vi "PingPong.BRAMStorage.vi"(5 "Bank 1":refnum<k21>, 6 "Line Status In":T2, 7 "Bank 0":refnum<k21>, 8 "BRAM Bank0 Write?":bool, 9 "Read Info":cluster{"Read Address":u16, "Read Valid":bool}, 10 "Write Info":cluster{"Write Address":u16, "Write Valid":bool}, 11 "Frame Data In":T3={"Pixel Data"=[0, 0, 0, 0], "Timestamps"={"Frame Timestamp"=0, "Acq Trigger Timestamp"=0, "Next Trigger Timestamp"=0}}) -> (0 "Output Valid":bool, 1 "Line Status Out":T2, 3 "Data Out":i16[](array[numeric]))   [LabVIEW 2014]
uses:
  Acquisition Engine/Acquisition Status.ctl
  <vilib>/rvi/DataTransferAndStorage/Container/Common/niFpgaContainerExecOnDevCompGetState.vi
  <vilib>/rvi/Emulation/niFpgaEmulationIsFPGAContextNoSignature.vi
  <vilib>/rvi/DataTransferAndStorage/Container/Common/niFpgaContainerGetUniqueNameForEmu.vi
  <vilib>/rvi/Emulation/niFpgaProcessEmulError.vi
  <vilib>/rvi/Emulation/niFpgaSctlEmulationGetInTimedLoop.vi
  <vilib>/rvi/errors/nirviReportUnexpectedCaseInternalError (U32).vi
  <vilib>/rvi/Memory/Memory_Emulation/niFpgaMemoryEmulationCacheClearOnFirstRun.vi
  <vilib>/rvi/Memory/Memory_Emulation/nirvimemoryEmulationManagerCache_MakeExclusive.vi
  <vilib>/rvi/Memory/Memory_Emulation/niFpgaMemoryEmulationValidateCache.vi
  <vilib>/rvi/Memory/Memory_Emulation/nirvimemoryEmulationManagerCache_InsertValue.vi
  <vilib>/Utility/error.llb/Clear Errors.vi
  <vilib>/rvi/Memory/Memory_Emulation/nirvimemoryEmulationManagerCache_ReleaseExclusive.vi
  <vilib>/rvi/Memory/Memory_Emulation/nirvimemoryEmulationManagerCache_GetValue.vi
  <vilib>/rvi/Memory/Memory_Emulation/nirvimemoryEmulationManagerCache_SetValue.vi
  <vilib>/rvi/Emulation/niFpgaSctlEmulationResourceMgr.vi
  <vilib>/rvi/DataTransferAndStorage/Container/XNode/niFpgaContainer.xnode
  <vilib>/rvi/Memory/Memory_Emulation/niFpgaMemoryEmulationRefIn.vi
panel:
  # "Copyright 2014 Vidrio Technologies\nScanImage 5 software is licensed under the Apache License, Version 2.0 (the \"License\"); you may not use any files contained\nwithin the ScanImage 5 release except in compliance with the License. You may obtain a copy of the License at\n http://www.apache.org/licenses/LICENSE-2.0\nUnless required by applicable law or agreed to in writing, software distributed under the License is distributed on an\n\"AS IS\" BASIS, WITHOUT WARRANTIES OR CONDITIONS OF ANY KIND, either express or implied. See the License for the\n specific language governing permissions and limitations under the License."
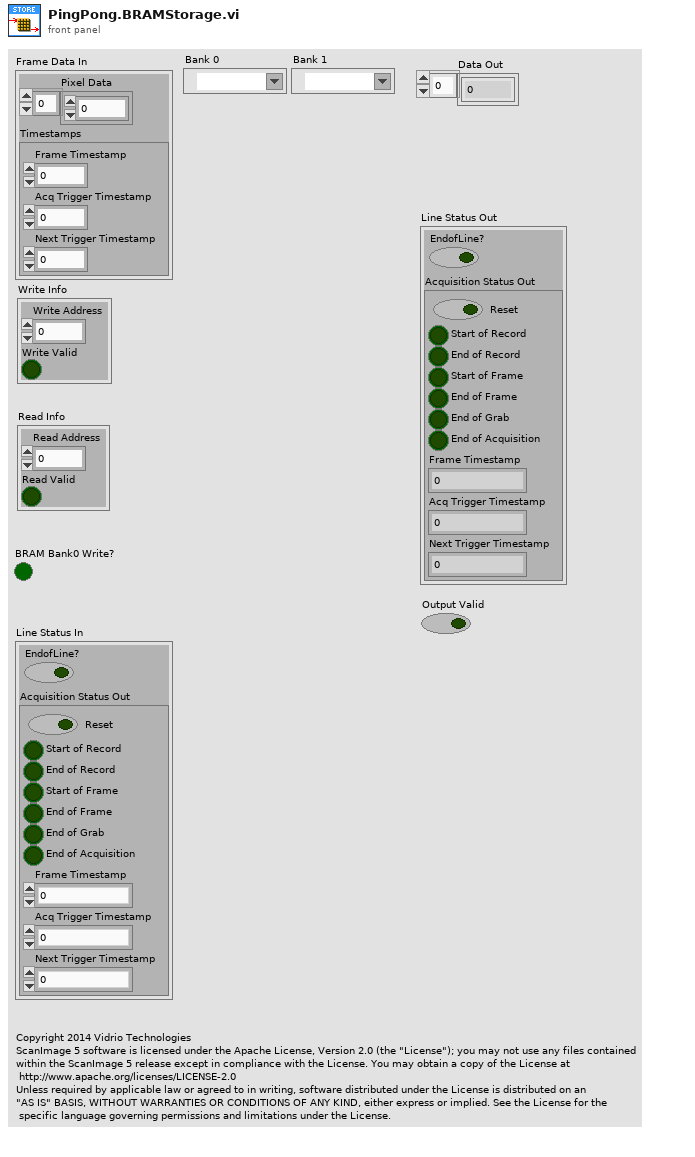
[diagram p1: front panel]
types:
  T1 = typedef "Acquisition Status.ctl" = cluster{"Reset":bool, "Start of Record":bool, "End of Record":bool, "Start of Frame":bool, "End of Frame":bool, "End of Grab":bool, "End of Acquisition":bool, "Frame Timestamp":u64, "Acq Trigger Timestamp":u64, "Next Trigger Timestamp":u64}
  T2 = cluster{"EndofLine?":bool, "Acquisition Status Out":T1}
  T3 = cluster{"Pixel Data":i16[], "Timestamps":cluster{"Frame Timestamp":u64, "Acq Trigger Timestamp":u64, "Next Trigger Timestamp":u64}}
  T4 = cluster{"Frame Timestamp":u64, "Acq Trigger Timestamp":u64, "Next Trigger Timestamp":u64}
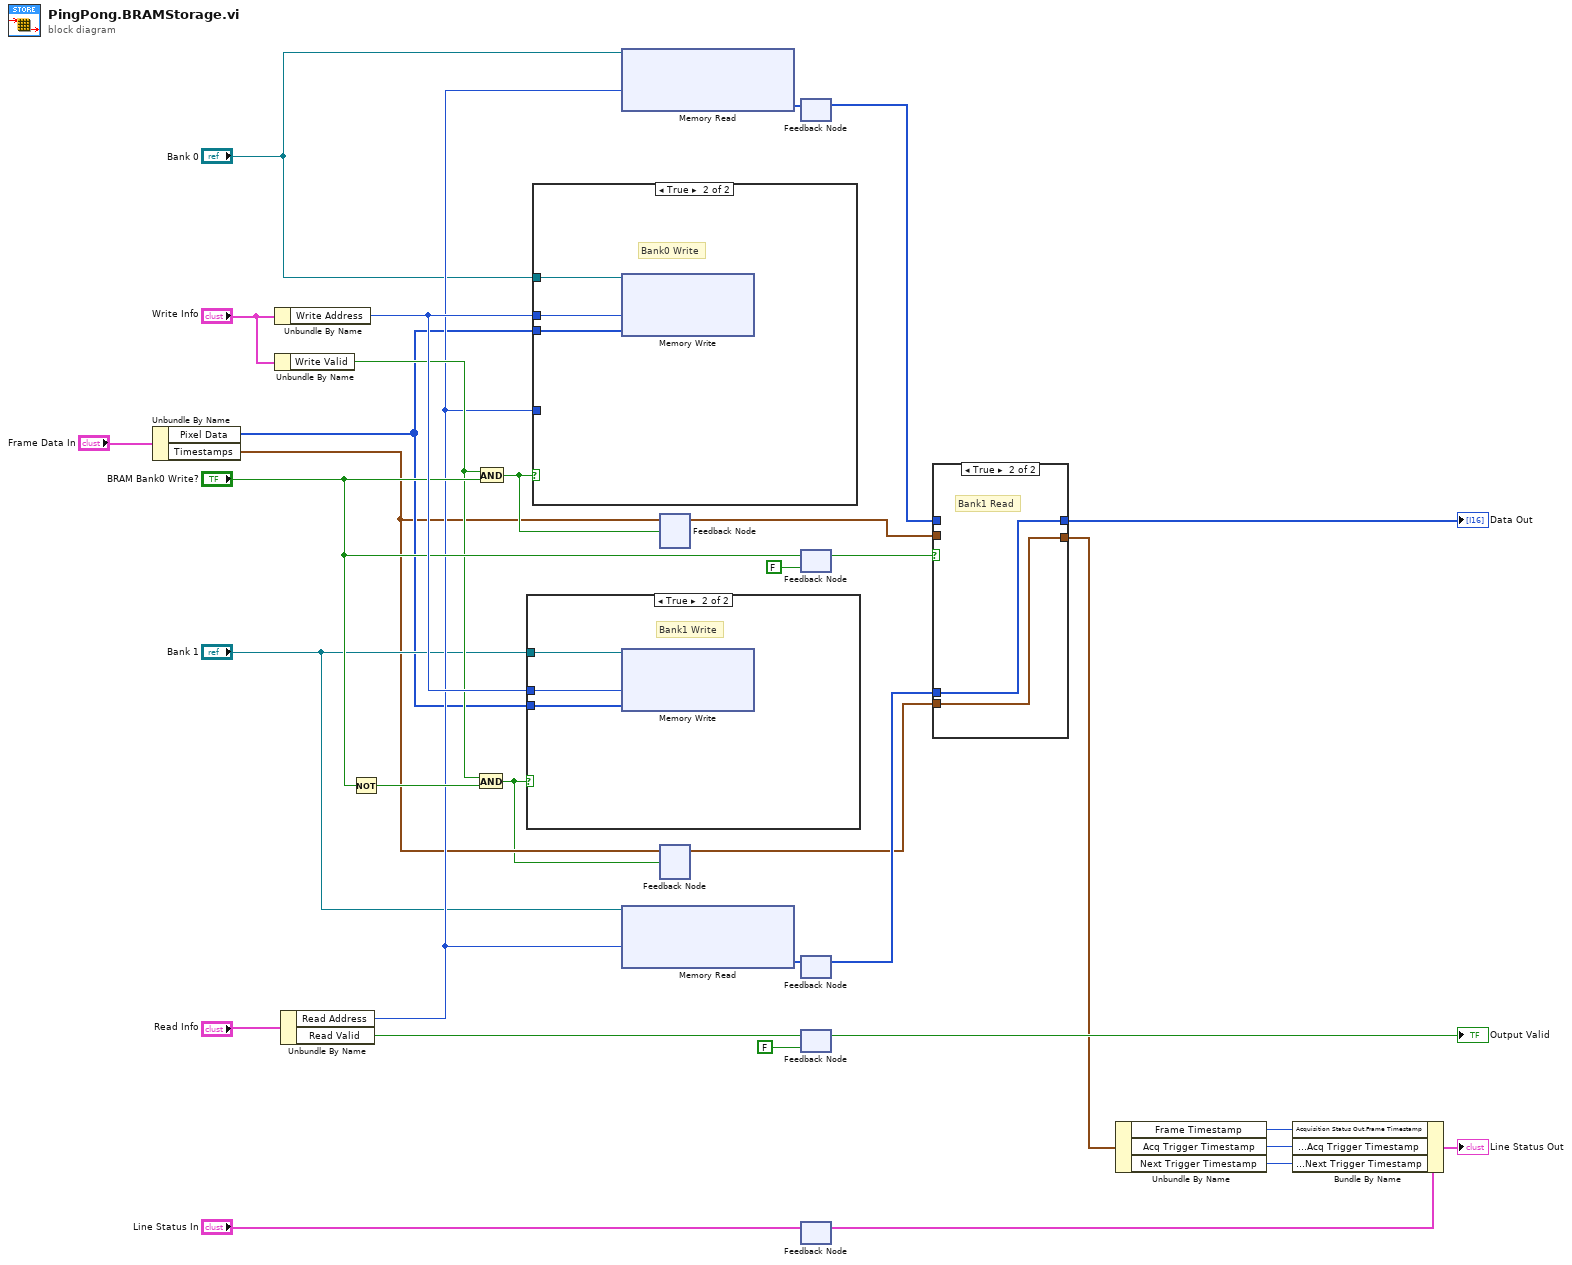
[diagram p0: block diagram]
diagram:
  n1 = Unbundle By Name("Frame Data In") -> ("Pixel Data"=w15:i16[], "Timestamps"=w12:T4)
  n2 = Unbundle By Name("Write Info") -> ("Write Address"=w32:u16)
  n3 = Unbundle By Name("Write Info") -> ("Write Valid"=w28:bool)
  n4 = Unbundle By Name("Read Info") -> ("Read Address"=w20:u16, "Read Valid"=w26:bool)
  n5 = Not(x="BRAM Bank0 Write?") -> (.not. x?=w31:bool)
  n6 = And(x=w28, y=w31) -> (x .and. y?=w9:bool)
  n7 = And(x=w28, y="BRAM Bank0 Write?") -> (x .and. y?=w13:bool)
  n8 = case shown="True" w9 {
    tunnel: "Bank 1" -> [_ w36]
    tunnel: w15 -> [_ w34]
    tunnel: w32 -> [_ w35]
    frame False {
    }
    frame True {
      # "Bank1 Write"
      n9 = xnode ("Memory Write")("Address"=w35, "Data"=w34, "Memory In"=w36) -> ()  [unwired: 1 out]
    }
  }
  n10 = case shown="True" w13 {
    tunnel: "Bank 0" -> [_ w39]
    tunnel: w32 -> [_ w38]
    tunnel: w15 -> [_ w37]
    tunnel: w20 -> [_ _]
    frame False {
      # "Bank0 Read"
    }
    frame True {
      # "Bank0 Write"
      n11 = xnode ("Memory Write")("Address"=w38, "Data"=w37, "Memory In"=w39) -> ()  [unwired: 1 out]
    }
  }
  n12 = xnode ("Memory Read")("Address"=w20, "Memory In"="Bank 0") -> ("Data"=w19:i16[])  [unwired: 1 out]
  n13 = xnode ("Memory Read")("Address"=w20, "Memory In"="Bank 1") -> ("Data"=w22:i16[])  [unwired: 1 out]
  n14 = feedback-in #1(w12, w13) -> ()
  n15 = feedback #1() -> (w11:T4)  [unwired: 1 in]
  n16 = feedback #2() -> (w10:T4)  [unwired: 1 in]
  n17 = feedback-in #2(w12, w9) -> ()
  n18 = feedback #3() -> (w18:i16[])  [unwired: 1 in]
  n19 = feedback-in #3(w19) -> ()
  n20 = feedback #4(FALSE ("BRAM Bank0 Write?")) -> (w27:bool)
  n21 = feedback-in #4("BRAM Bank0 Write?") -> ()
  n22 = feedback #5() -> (w21:i16[])  [unwired: 1 in]
  n23 = feedback-in #5(w22) -> ()
  n24 = feedback-in #6(w26) -> ()
  n25 = feedback #6(FALSE ("Read Valid")) -> (→"Output Valid":bool)
  n26 = feedback #7() -> (w7:T2)  [unwired: 1 in]
  n27 = feedback-in #7("Line Status In") -> ()
  n28 = case shown="True" w27 {
    tunnel: w18 -> [w41 _]
    tunnel: w21 -> [_ w43]
    tunnel: [w41 w43] -> w8
    tunnel: w11 -> [w40 _]
    tunnel: w10 -> [_ w42]
    tunnel: [w40 w42] -> w5
    frame False {
      # "Bank0 Read"
    }
    frame True {
      # "Bank1 Read"
    }
  }
  "Data Out" <- w8
  n29 = Unbundle By Name(w5) -> ("Frame Timestamp"=w4:u64, "Acq Trigger Timestamp"=w3:u64, "Next Trigger Timestamp"=w1:u64)
  n30 = Bundle By Name(cluster=w7, "Acquisition Status Out.Frame Timestamp"=w4, "Acquisition Status Out.Acq Trigger Timestamp"=w3, "Acquisition Status Out.Next Trigger Timestamp"=w1) -> (→"Line Status Out":T2)
